vi "TP program.vi"(3 "error in (no error)":errorcluster, 5 "Program path":path) -> (0 "error out":errorcluster, 1 ".not. x?":bool, 2 "order":string caption="FileName:")   [LabVIEW 2018]
panel:
  out "Row":i32
  out "文件数组":string[][](array[string])
  out "大小":i32
  out "exit":bool
  in  "Bar":bool
  in  "Cancel":bool
  in  "OK":bool
  in  "Program list":i32(listbox)
  # "TestProgramSelet"
  # "C:\\Users\\Administrator\\Desktop\\ATE_Program\\ModelInformation"
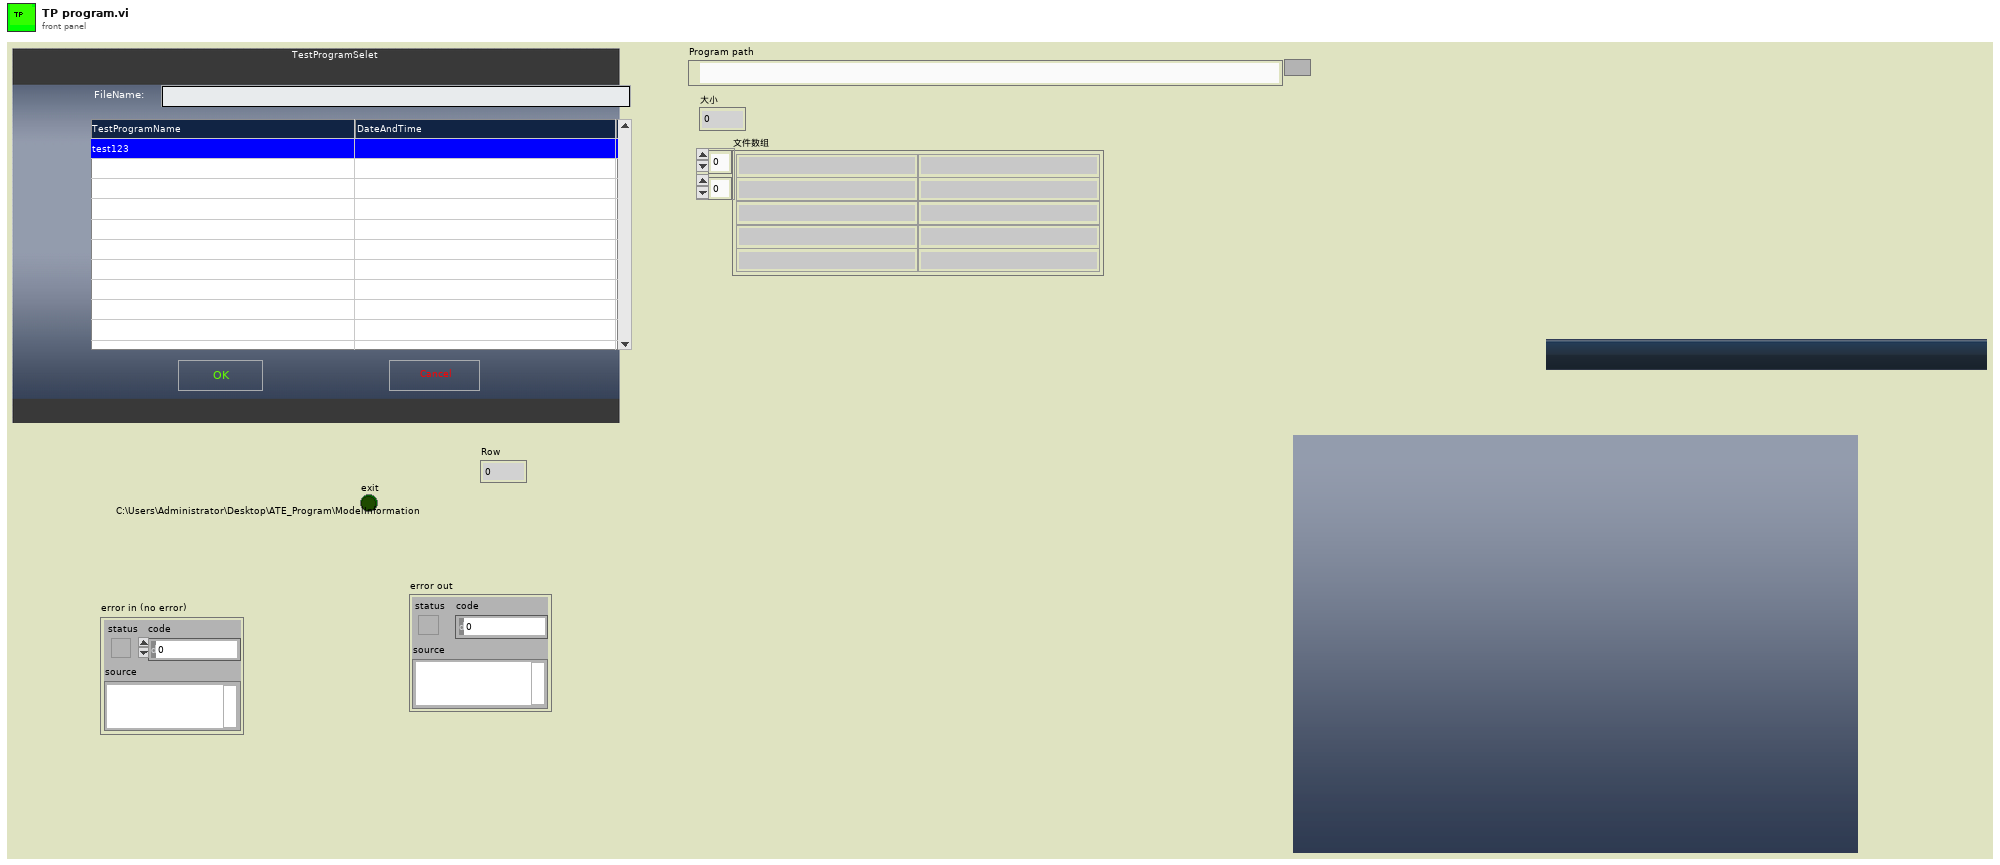
[diagram p1: front panel]
types:
  T1 = typedef "Window Refnum.ctl" = refnum<k1>
  T2 = typedef "Window Rectangle.ctl" = cluster{"left":i16, "top":i16, "right":i16, "bottom":i16}
  T3 = typedef "LVPoint32TypeDef.ctl" = cluster{"Horizontal":i32, "Vertical":i32}
  T4 = typedef "LVRowAndColumnTypeDef.ctl" = cluster{"Row":i32, "Column":i32}
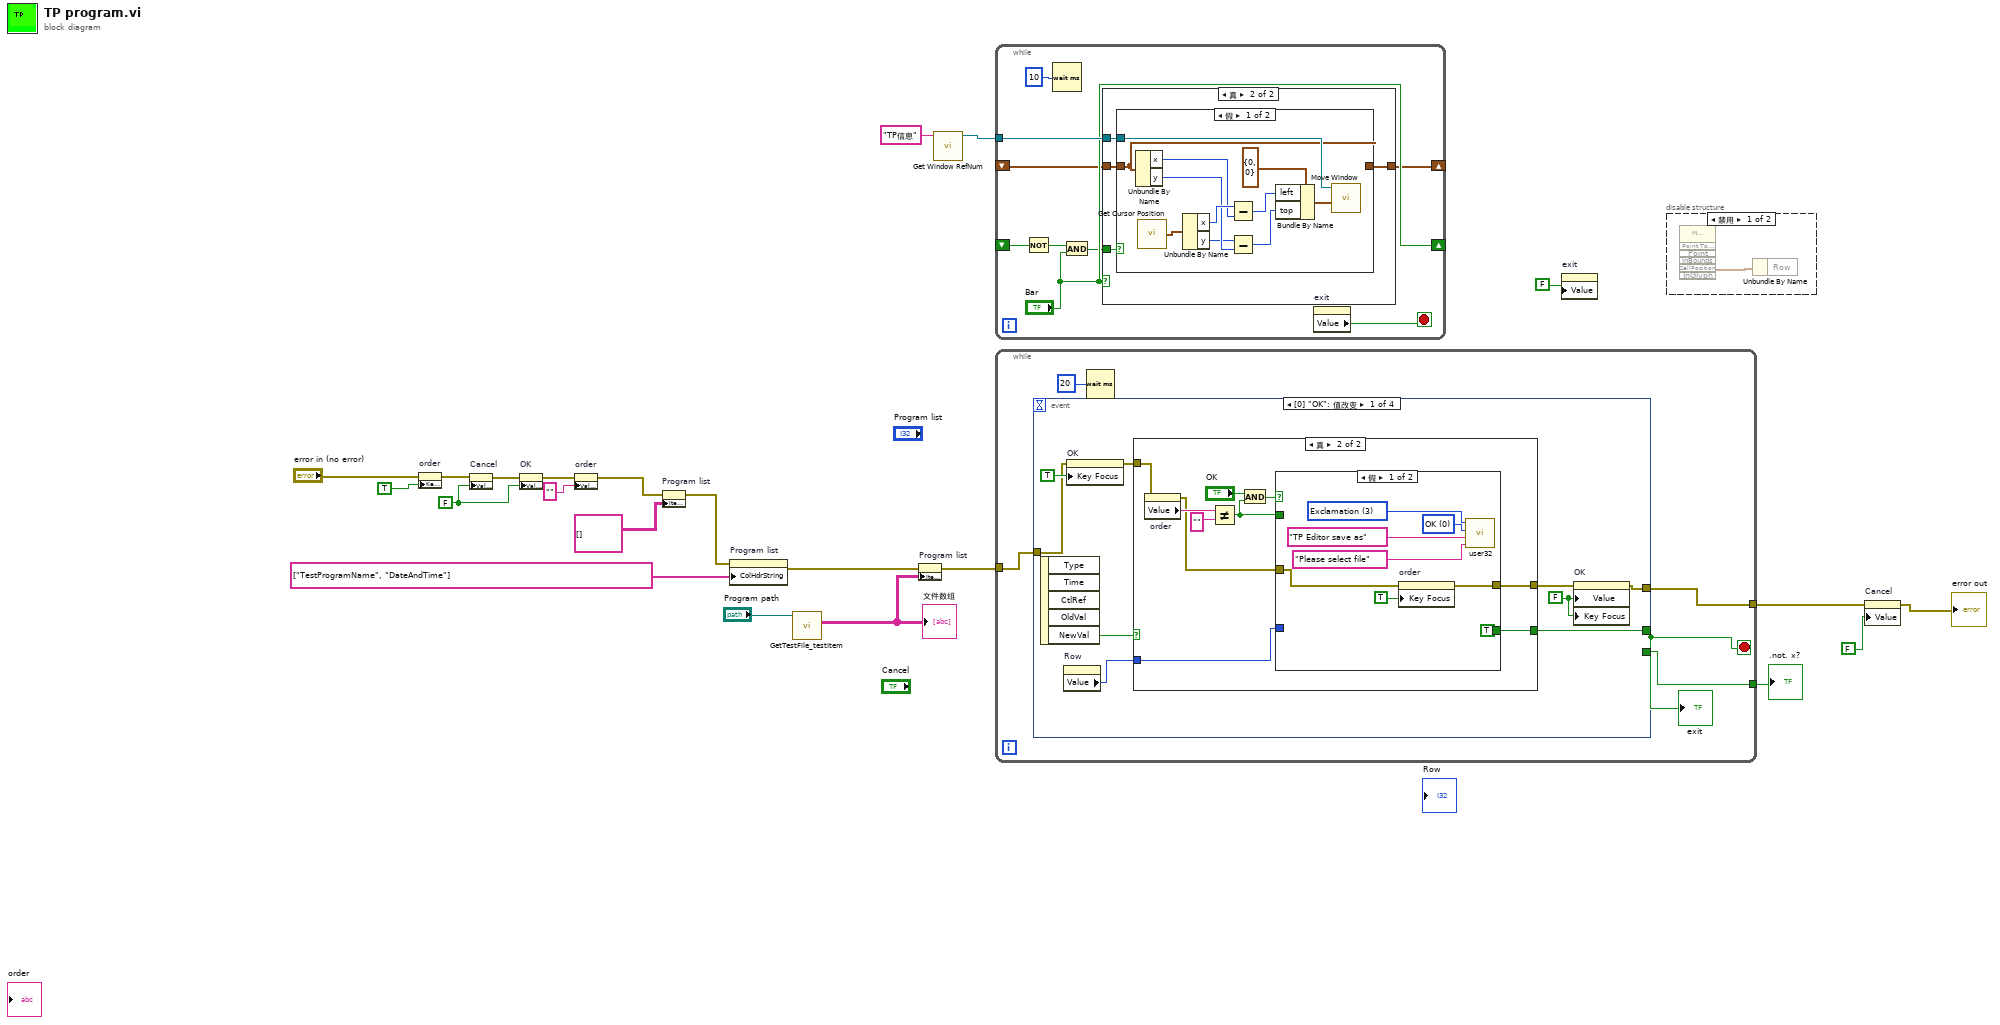
[diagram p0: block diagram]
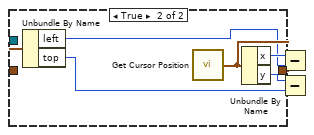
[diagram p4: hidden frame]
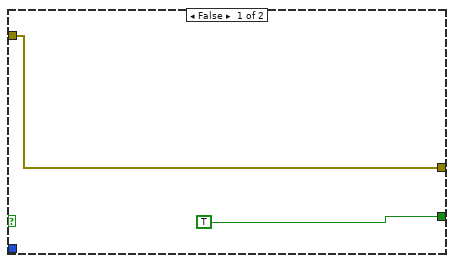
[diagram p5: hidden frame]
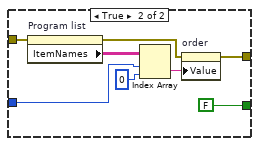
[diagram p6: hidden frame]
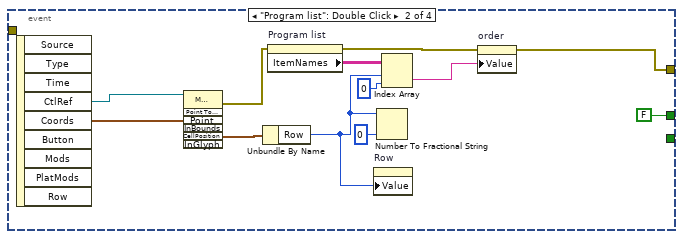
[diagram p7: hidden frame]
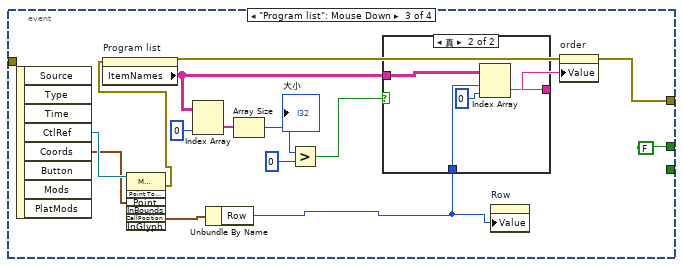
[diagram p8: hidden frame]
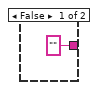
[diagram p9: hidden frame]
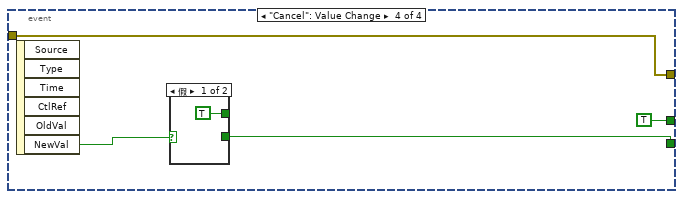
[diagram p10: hidden frame]
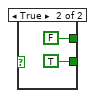
[diagram p11: hidden frame]
diagram:
  w16 = FALSE
  n1 = property on="order" class="Str"(error in="error in (no error)", "Key Focus"=TRUE) -> (error out=w2:errorcluster)  [unwired: 1 in, 1 out]
  n2 = property on="Cancel" class="Bool"(error in=w2, "Value"=w16) -> (error out=w17:errorcluster)  [unwired: 1 in, 1 out]
  n3 = property on="OK" class="Bool"(error in=w17, "Value"=w16) -> (error out=w18:errorcluster)  [unwired: 1 in, 1 out]
  n4 = property on="order" class="Str"(error in=w18, "Value"="") -> (error out=w3:errorcluster)  [unwired: 1 in, 1 out]
  n5 = property on="Program list" class="MCListbox (严格)"(error in=w3, "ItemNames"=string[][] []) -> (error out=w7:errorcluster)  [unwired: 1 in, 1 out]
  n6 = property on="Program list" class="MCListbox (严格)"(error in=w7, "ColHdrString"=string[] ["TestProgramName", "DateAndTime"] ("Column Header Strings[]")) -> (error out=w5:errorcluster)  [unwired: 1 in, 1 out]
  n7 = call "GetTestFile_testItem.vi"("Program path"="Program path") -> ("转置的数组"=w6:string[][])  [unwired: 9 in, 1 out]
  "文件数组" <- w6
  n8 = property on="Program list" class="MCListbox (严格)"(error in=w5, "ItemNames"=w6) -> (error out=w4:errorcluster)  [unwired: 1 in, 1 out]
  n9 = call "Get Window RefNum.vi"("window name (\"\")"="TP信息" ("window name (\"\")")) -> ("window refnum (NaWR)"=w10:T1)  [unwired: 1 in, 7 out]
  n10 = while {
    shift-left: _ -> [w25]
    shift-right: [w26] -> _
    shift-left: _ -> [w29]
    shift-right: ["Bar"] -> _
    tunnel: w10 -> [w30]
    stop <- w23 stop-if-true
    n11 = Not(x=w29) -> (.not. x?=w28:bool)
    n12 = Wait (ms)(milliseconds to wait=u32 10) -> ()  [unwired: 1 out]
    n13 = And(x=w28, y="Bar") -> (x .and. y?=w24:bool)
    n14 = case shown="真" "Bar" {
      tunnel: w30 -> [_ w36]
      tunnel: [w32 w35] -> w26
      tunnel: w25 -> [w32 w33]
      tunnel: w24 -> [_ w34]
      frame False {
      }
      frame True {
        n15 = case shown="假" w34 {
          tunnel: w36 -> [w42 w58]
          tunnel: [w37 w48] -> w35
          tunnel: w33 -> [w37 _]
          frame False {
            n16 = Unbundle By Name(w37) -> ("x"=w45:i16, "y"=w44:i16)
            n17 = call "Get Cursor Position.vi"() -> ("cursor position"=w47:cluster{"x":i16, "y":i16})
            n18 = Unbundle By Name(w47) -> ("x"=w46:i16, "y"=w43:i16)
            n19 = Subtract(x=w46, y=w45) -> (x-y=w39:i16)
            n20 = Subtract(x=w43, y=w44) -> (x-y=w40:i16)
            n21 = Bundle By Name(cluster=cluster{"left":i16, "top":i16} {"left"=0, "top"=0} ("new position (0,0)"), "left"=w39, "top"=w40) -> (w38:cluster{"left":i16, "top":i16})
            n22 = call "Move Window.vi"("new position (0,0)"=w38, "window refnum (NaWR)"=w42) -> ()  [unwired: 2 in, 4 out]
          }
          frame True {
            n23 = call "Get Window Rectangle.vi"("window refnum (NaWR)"=w58) -> ("window rect"=w57:T2)  [unwired: 1 in, 5 out]
            n24 = call "Extract Window Origin.vi"("window rect"=w57) -> ("window origin"=w56:cluster{"left":i16, "top":i16})  [unwired: 1 out]
            n25 = Unbundle By Name(w56) -> ("left"=w53:i16, "top"=w52:i16)
            n26 = call "Get Cursor Position.vi"() -> ("cursor position"=w55:cluster{"x":i16, "y":i16})
            n27 = Unbundle By Name(w55) -> ("x"=w54:i16, "y"=w51:i16)
            n28 = Subtract(x=w54, y=w53) -> (x-y=w49:i16)
            n29 = Subtract(x=w51, y=w52) -> (x-y=w50:i16)
            n30 = Bundle By Name(cluster=w55, "x"=w49, "y"=w50) -> (w48:cluster{"x":i16, "y":i16})
          }
        }
      }
    }
    n31 = property on="exit" class="Bool (严格)"() -> ("Value"=w23:bool)  [unwired: 2 in, 2 out]
  }
  n32 = while {
    tunnel: [w63] -> w15
    tunnel: [w62] -> w12
    tunnel: w4 -> [w61]
    stop <- w59 stop-if-true
    n33 = event shown="[0] \"OK\": 值改变" {
      selector: _ -> [_ _ _ _]
      dyn-events: _ -> [_ _ _ _]
      timeout: _ -> [_ _ _ _]
      tunnel: [w72 FALSE FALSE TRUE] -> w59
      tunnel: [_ _ _ w135] -> w63
      tunnel: [w66 w111 w125 w134] -> w62
      tunnel: w61 -> [w65 _ _ w134]
      event "OK": Value Change {
        w70 = FALSE
        n34 = event-data() -> ("NewVal"=w69:bool)  [unwired: 5 out]
        n35 = property on="Row" class="DigNum (严格)"() -> ("Value"=w64:i32)  [unwired: 2 in, 2 out]
        n36 = property on="OK" class="Bool"(error in=w65, "Key Focus"=TRUE) -> (error out=w67:errorcluster)  [unwired: 1 in, 1 out]
        n37 = case shown="真" w69 {
          tunnel: [TRUE w79] -> w72
          tunnel: [w73 w78] -> w71
          tunnel: w67 -> [w73 w77]
          tunnel: w64 -> [_ w75]
          frame False {
          }
          frame True {
            n38 = property on="order" class="Str"(error in=w77) -> (error out=w76:errorcluster, "Value"=w84:string)  [unwired: 1 in, 1 out]
            n39 = Not Equal?(x=w84, y="") -> (x != y?=w80:bool)
            n40 = And(x="OK", y=w80) -> (x .and. y?=w82:bool)
            n41 = case shown="假" w82 {
              tunnel: [TRUE FALSE] -> w79
              tunnel: w80 -> [_ _]
              tunnel: [w86 w96] -> w78
              tunnel: w76 -> [w85 w95]
              tunnel: w75 -> [_ w93]
              frame False {
                w90 = u16 0 items=["OK", "OK+Cancel", "Abort+Retry+Ignore", "Yes+ON+Cancel", "Yes+No", "Retry+Cancel", "Cancel+Retry+Continue"] ("Buttons")
                w91 = u16 3 items=["None", "Critical", "Question", "Exclamation", "Infomation"] ("Icon")
                n42 = property on="order" class="Str"(error in=w85, "Key Focus"=TRUE) -> (error out=w86:errorcluster)  [unwired: 1 in, 1 out]
                n43 = call "user32.vi"("Icon"=w91, "Buttons"=w90, "Ipcaption"="TP Editor save as", "IP Text"="Please select file") -> ()  [unwired: 2 out]
              }
              frame True {
                n44 = property on="Program list" class="MCListbox (严格)"(error in=w95) -> (error out=w94:errorcluster, "ItemNames"=w99:string[][])  [unwired: 1 in, 1 out]
                n45 = Index Array(array=w99, index (row)=w93, index (col)=0 ("disabled index (col)")) -> (element=w97:string)
                n46 = property on="order" class="Str"(error in=w94, "Value"=w97) -> (error out=w96:errorcluster)  [unwired: 1 in, 1 out]
              }
            }
          }
        }
        n47 = property on="OK" class="Bool"(error in=w71, "Value"=w70, "Key Focus"=w70) -> (error out=w66:errorcluster)  [unwired: 1 in, 1 out]
      }
      event "Program list": Double Click {
        n48 = event-data() -> ("CtlRef"=w110:refnum<vi>, "Coords"=w109:T3)  [unwired: 8 out]
        n49 = invoke class="MCListbox (严格)" method="Point To Row Column"(reference=w110, "Point"=w109) -> (error out=w102:errorcluster, "CellPosition"=w108:T4)  [unwired: 5 in, 5 out]
        n50 = Unbundle By Name(w108) -> ("Row"=w101:i32)
        n51 = property on="Program list" class="MCListbox (严格)"(error in=w102) -> (error out=w104:errorcluster, "ItemNames"=w107:string[][])  [unwired: 1 in, 1 out]
        n52 = property on="Row" class="DigNum (严格)"("Value"=w101) -> ()  [unwired: 2 in, 2 out]
        n53 = Number To Fractional String(number=w101, precision (6)=i16 0 ("精度(6)")) -> ()  [unwired: 2 in, 1 out]
        n54 = Index Array(array=w107, index (row)=w101, index (col)=0 ("disabled index (col)")) -> (element=w105:string)
        n55 = property on="order" class="Str"(error in=w104, "Value"=w105) -> (error out=w111:errorcluster)  [unwired: 1 in, 1 out]
      }
      event "Program list": Mouse Down {
        n56 = event-data() -> ("CtlRef"=w116:refnum<vi>, "Coords"=w115:T3)  [unwired: 7 out]
        n57 = invoke class="MCListbox (严格)" method="Point To Row Column"(reference=w116, "Point"=w115) -> (error out=w114:errorcluster, "CellPosition"=w117:T4)  [unwired: 5 in, 5 out]
        n58 = property on="Program list" class="MCListbox (严格)"(error in=w114) -> (error out=w124:errorcluster, "ItemNames"=w123:string[][])  [unwired: 1 in, 1 out]
        n59 = Index Array(array=w123, index (col)=0 ("禁用的索引 (列)")) -> (element=w121:string[])  [unwired: 1 in]
        n60 = Unbundle By Name(w117) -> ("Row"=w113:i32)
        n61 = Array Size(array=w121) -> (size(s)=w120:i32)
        "大小" <- w120
        n62 = Greater?(x=w120, y=0) -> (0:w118:bool)
        n63 = case shown="真" w118 {
          tunnel: ["" w131] -> w127
          tunnel: w123 -> [_ w130]
          tunnel: w113 -> [_ w129]
          frame False {
          }
          frame True {
            n64 = Index Array(array=w130, index (row)=w129, index (col)=0 ("disabled index (col)")) -> (element=w131:string)
          }
        }
        n65 = property on="Row" class="DigNum (严格)"("Value"=w113) -> ()  [unwired: 2 in, 2 out]
        n66 = property on="order" class="Str"(error in=w124, "Value"=w127) -> (error out=w125:errorcluster)  [unwired: 1 in, 1 out]
      }
      event "Cancel": Value Change {
        n67 = event-data() -> ("NewVal"=w136:bool)  [unwired: 6 out]
        n68 = case shown="假" w136 {
          tunnel: [TRUE FALSE] -> _
          tunnel: [_ TRUE] -> w135
          frame False {
          }
          frame True {
          }
        }
      }
    }
    "exit" <- w59
    n69 = Wait (ms)(milliseconds to wait=u32 20) -> ()  [unwired: 1 out]
  }
  ".not. x?" <- w15
  n70 = property on="exit" class="Bool (严格)"("Value"=FALSE (".not. x?")) -> ()  [unwired: 2 in, 2 out]
  n71 = disable-structure shown="禁用" {
    frame Disabled {
      n72 = invoke class="MCListbox (严格)" method="Point To Row Column"() -> ("CellPosition"=w140:T4)  [unwired: 6 in, 7 out]
      n73 = Unbundle By Name(w140) -> ()  [unwired: 1 out]
    }
    frame Enabled {
    }
  }
  n74 = property on="Cancel" class="Bool"(error in=w12, "Value"=FALSE) -> (error out=→"error out":errorcluster)  [unwired: 1 in, 1 out]
